vi "CAN Get List File Msg.vi"(8 "error in (no error)":errorcluster, 9 "pCANMsg":T1, 10 "MsgLen":i32, 11 "MsgIndex":i32) -> (0 "error out":errorcluster, 1 "pCANMsg out":T1, 3 "function return":i32)   [LabVIEW 2010, in "usb2an.lvlib"]
doc: "int WINAPI CAN_GetListFileMsg(int MsgIndex,int MsgLen,CAN_MSG *pCANMsg);"
uses:
  usb2an.lvlib
  USB2XXX.dll
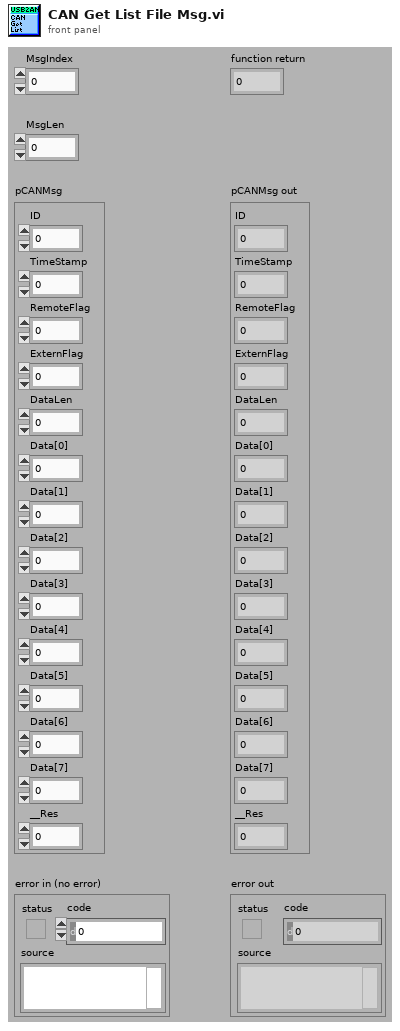
[diagram p1: front panel]
types:
  T1 = cluster{"ID":u32, "TimeStamp":u32, "RemoteFlag":u8, "ExternFlag":u8, "DataLen":u8, "Data[0]":u8, "Data[1]":u8, "Data[2]":u8, "Data[3]":u8, "Data[4]":u8, "Data[5]":u8, "Data[6]":u8, "Data[7]":u8, "__Res":u8}
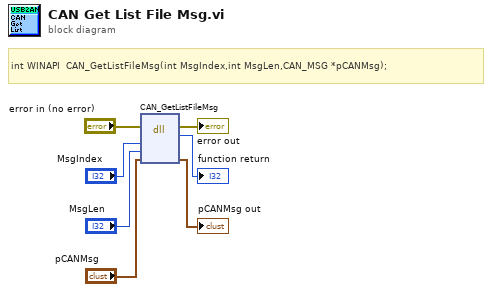
[diagram p0: block diagram]
diagram:
  # "int WINAPI  CAN_GetListFileMsg(int MsgIndex,int MsgLen,CAN_MSG *pCANMsg);"
  n1 = dll-call lib="E:/OtherWork/STM32/USB2XXX_Example/sdk/api/Labview/USB2XXX.*" fn="CAN_GetListFileMsg"(error in="error in (no error)", "MsgIndex"="MsgIndex", "MsgLen"="MsgLen", "pCANMsg"="pCANMsg") -> (error out=→"error out":errorcluster, →"function return":i32, "pCANMsg"=→"pCANMsg out":T1)  [unwired: 4 in, 1 out]
